vi "Read Counter.vi"(8 "error in (no error)":errorcluster, 11 "VISA resource name":refnum<visa-resource-name>) -> (0 "error out":errorcluster, 2 "Deposit Counter":i32, 3 "VISA resource name out":refnum<visa-resource-name>)   [LabVIEW 2020, in "EFD Ultimus V.lvlib"]
doc: "Reads the current seven digit deposit count that is stored in the dispenser"
uses:
  EFD Ultimus V.lvlib
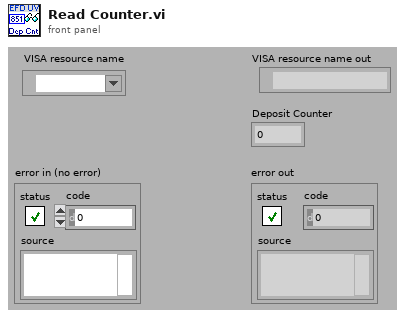
[diagram p1: front panel]
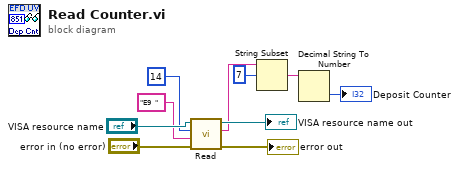
[diagram p0: block diagram]
diagram:
  n1 = call "Read.vi"("error in (no error)"="error in (no error)", "Command To Write"="E9  ", "Bytes to Read (11)"=u32 14 ("Bytes to Read"), "VISA resource name"="VISA resource name") -> ("error out"=→"error out":errorcluster, "Ultimus V Feedback Data"=w5:string, "VISA resource name out"=→"VISA resource name out":refnum<visa-resource-name>)  [unwired: 5 out]
  n2 = String Subset(string=w5, offset (0)=7) -> (substring=w4:string)  [unwired: 1 out]
  n3 = Decimal String To Number(string=w4) -> (number=→"Deposit Counter":i32)  [unwired: 3 out]
